vi "Errors.vi"   [LabVIEW 2017, in "Data Sharing Framework Engine.lvlib" / "Memory Buffer.lvclass"]
uses:
  Memory Buffer.lvclass
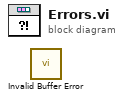
[diagram p0: block diagram]
diagram:
  n1 = call "Invalid Buffer Error.vi"() -> ()  [unwired: 10 in, 2 out]
